vi "Example_LowLevelImage.vi"() -> ()   [LabVIEW 2019, in "LcPictureBox.lvclass"]
uses:
  LcPictureBox.lvclass
  System.Windows.Forms
  System.Drawing
panel:
  in  "PictureBox 1":refnum<k24>(container)
  out "Error Out":errorcluster
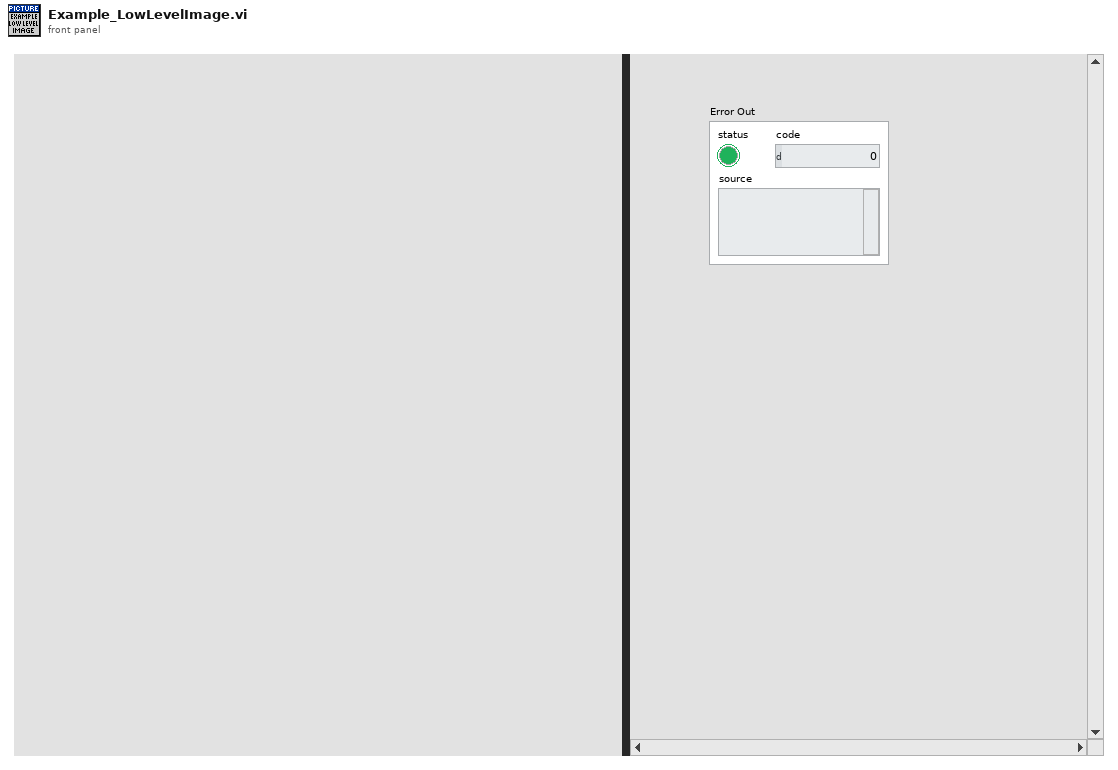
[diagram p1: front panel]
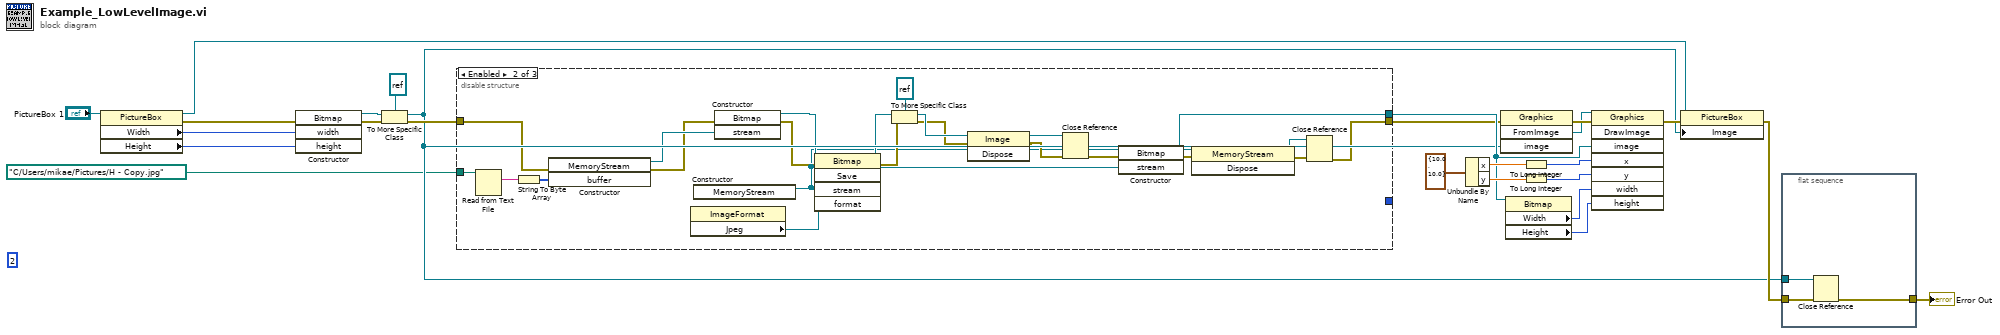
[diagram p0: block diagram]
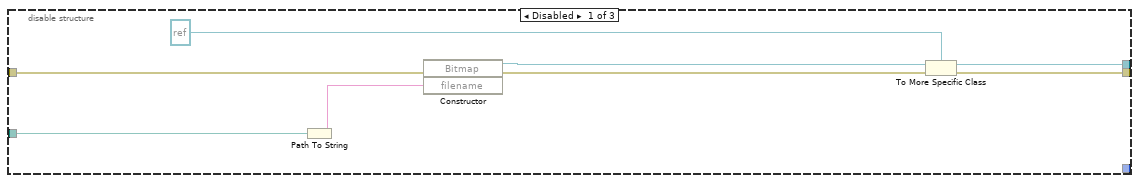
[diagram p2: hidden frame]
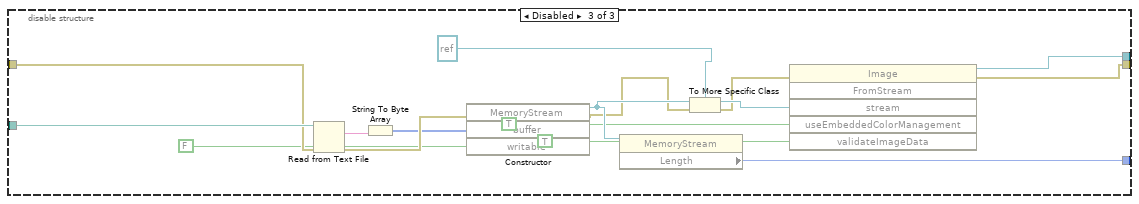
[diagram p3: hidden frame]
diagram:
  (unwired) 2
  n1 = property on="Property Node" class="PictureBox"(reference="PictureBox 1") -> (reference out=w5:refnum<k24>, error out=w8:errorcluster, "Width"=w18:i32, "Height"=w17:i32)  [unwired: 1 in]
  n2 = constructor class="Bitmap"(error in=w8, "width"=w18, "height"=w17) -> (reference out=w21:refnum<k24>, error out=w20:errorcluster)  [unwired: 2 in, 3 out]
  n3 = To More Specific Class(target class=refnum<k24> refnum, reference=w21, error in=w20) -> (specific class reference=w2:refnum<k24>, error out=w12:errorcluster)
  n4 = disable-structure shown="Enabled" {
    disable-tunnel: [w29 w40 w71] -> w15
    disable-tunnel: [w28 w41 w70] -> w13
    disable-tunnel: w12 -> [w27 w34 w68]
    disable-tunnel: path "C:/Users/mikae/Pictures/H - Copy.jpg" ("path (use dialog)") -> [w26 w39 w72]
    disable-tunnel: [_ _ w59] -> _
    frame Disabled {
      n5 = Path To String(path=w26) -> (string=w30:string)
      n6 = constructor class="Bitmap"(error in=w27, "filename"=w30) -> (reference out=w32:refnum<k24>, error out=w31:errorcluster)  [unwired: 2 in, 2 out]
      n7 = To More Specific Class(target class=refnum<k24> refnum, reference=w32, error in=w31) -> (specific class reference=w29:refnum<k24>, error out=w28:errorcluster)
    }
    frame Enabled {
      n8 = Read from Text File(file (use dialog)=w39) -> (text=w38:string)  [unwired: 3 in, 3 out]
      n9 = String To Byte Array(string=w38) -> (unsigned byte array=w37:u8[])
      n10 = constructor class="MemoryStream"(error in=w34, "buffer"=w37) -> (reference out=w36:refnum<k24>, error out=w35:errorcluster)  [unwired: 2 in, 2 out]
      n11 = property class="ImageFormat"() -> ("Jpeg"=w52:refnum<k24>)  [unwired: 2 in, 2 out]
      n12 = constructor class="MemoryStream"() -> (reference out=w45:refnum<k24>)  [unwired: 3 in, 2 out]
      n13 = constructor class="Bitmap"(error in=w35, "stream"=w36) -> (reference out=w50:refnum<k24>, error out=w48:errorcluster)  [unwired: 2 in, 2 out]
      n14 = invoke class="Bitmap" method="Save"(reference=w50, error in=w48, "stream"=w45, "format"=w52) -> (reference out=w49:refnum<k24>, error out=w47:errorcluster)  [unwired: 1 in, 3 out]
      n15 = To More Specific Class(target class=refnum<k24> refnum, reference=w49, error in=w47) -> (specific class reference=w55:refnum<k24>, error out=w51:errorcluster)
      n16 = invoke class="Image" method="Dispose"(reference=w55, error in=w51) -> (reference out=w54:refnum<k24>, error out=w53:errorcluster)  [unwired: 1 in, 1 out]
      n17 = Close Reference(reference=w54, error in (no error)=w53) -> (error out=w42:errorcluster)
      n18 = constructor class="Bitmap"(error in=w42, "stream"=w45) -> (reference out=w40:refnum<k24>, error out=w46:errorcluster)  [unwired: 2 in, 2 out]
      n19 = invoke class="MemoryStream" method="Dispose"(reference=w45, error in=w46) -> (reference out=w43:refnum<k24>, error out=w44:errorcluster)  [unwired: 1 in, 1 out]
      n20 = Close Reference(reference=w43, error in (no error)=w44) -> (error out=w41:errorcluster)
    }
    frame Disabled {
      n21 = Read from Text File(file (use dialog)=w72, error in=w68) -> (text=w67:string, error out=w69:errorcluster)  [unwired: 2 in, 2 out]
      n22 = String To Byte Array(string=w67) -> (unsigned byte array=w66:u8[])
      n23 = constructor class="MemoryStream"(error in=w69, "buffer"=w66, "writable"=FALSE) -> (reference out=w64:refnum<k24>, error out=w61:errorcluster)  [unwired: 2 in, 3 out]
      n24 = property class="MemoryStream"(reference=w64) -> ("Length"=w59:i64)  [unwired: 1 in, 2 out]
      n25 = To More Specific Class(target class=refnum<k24> refnum ("stream"), reference=w64, error in=w61) -> (specific class reference=w62:refnum<k24>, error out=w60:errorcluster)
      n26 = invoke class="Image" method="FromStream"(error in=w60, "stream"=w62, "useEmbeddedColorManagement"=TRUE, "validateImageData"=TRUE) -> (reference out=w71:refnum<k24>, error out=w70:errorcluster)  [unwired: 2 in, 4 out]
    }
  }
  n27 = Unbundle By Name(cluster{"x":sgl, "y":sgl} {"x"=10.0, "y"=10.0} ("input cluster")) -> ("x"=w25:sgl, "y"=w24:sgl)
  n28 = invoke class="Graphics" method="FromImage"(error in=w13, "image"=w2) -> (error out=w14:errorcluster, "FromImage"=w7:refnum<k24>)  [unwired: 2 in, 2 out]
  n29 = property class="Bitmap"(reference=w15) -> ("Width"=w10:i32, "Height"=w9:i32)  [unwired: 1 in, 2 out]
  n30 = To Long Integer(number=w25) -> (32bit integer=w23:i32)
  n31 = To Long Integer(number=w24) -> (32bit integer=w22:i32)
  n32 = invoke class="Graphics" method="DrawImage"(reference=w7, error in=w14, "image"=w15, "x"=w23, "y"=w22, "width"=w10, "height"=w9) -> (error out=w6:errorcluster)  [unwired: 1 in, 7 out]
  n33 = property class="PictureBox"(reference=w5, error in=w6, "Image"=w2) -> (error out=w4:errorcluster)  [unwired: 1 out]
  n34 = flat-sequence {
    tunnel: w4 -> [w75]
    tunnel: [w74] -> w3
    tunnel: w2 -> [w73]
    frame #0 {
      n35 = Close Reference(reference=w73, error in (no error)=w75) -> (error out=w74:errorcluster)
    }
  }
  "Error Out" <- w3
